vi "Read (Transient).vi"(8 "error in (no error)":errorcluster, 11 "VISA resource name":refnum<visa-resource-name>) -> (0 "error out":errorcluster, 1 "Peak-to-Peak":dbl, 2 "Measurement":dbl, 3 "VISA resource name out":refnum<visa-resource-name>, 5 "Minimum":dbl, 7 "Maximum":dbl)   [LabVIEW 2020, in "Agilent 34401.lvlib"]
doc: "Starts a new single reading and returns the measurement, transient maximum, transient minimum, and peak-to-peak values.\n\n<B>Note:</B>\n\n(1) This VI only applies to the 34410/34411 models. \n\n(2) This VI only supports DC/AC current and voltage measurements."
uses:
  <instrlib>/Agilent 34401/Agilent 34401.lvlib
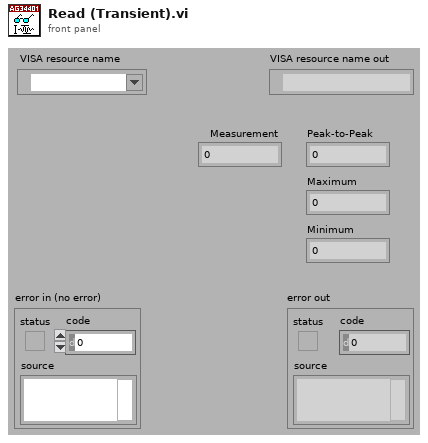
[diagram p1: front panel]
types:
  T1 = typedef "Agilent 34401.lvlib/Extended User Data.ctl" = cluster{"Trigger Source":u16, "Math Storage":u16, "Agilent Model":i32}
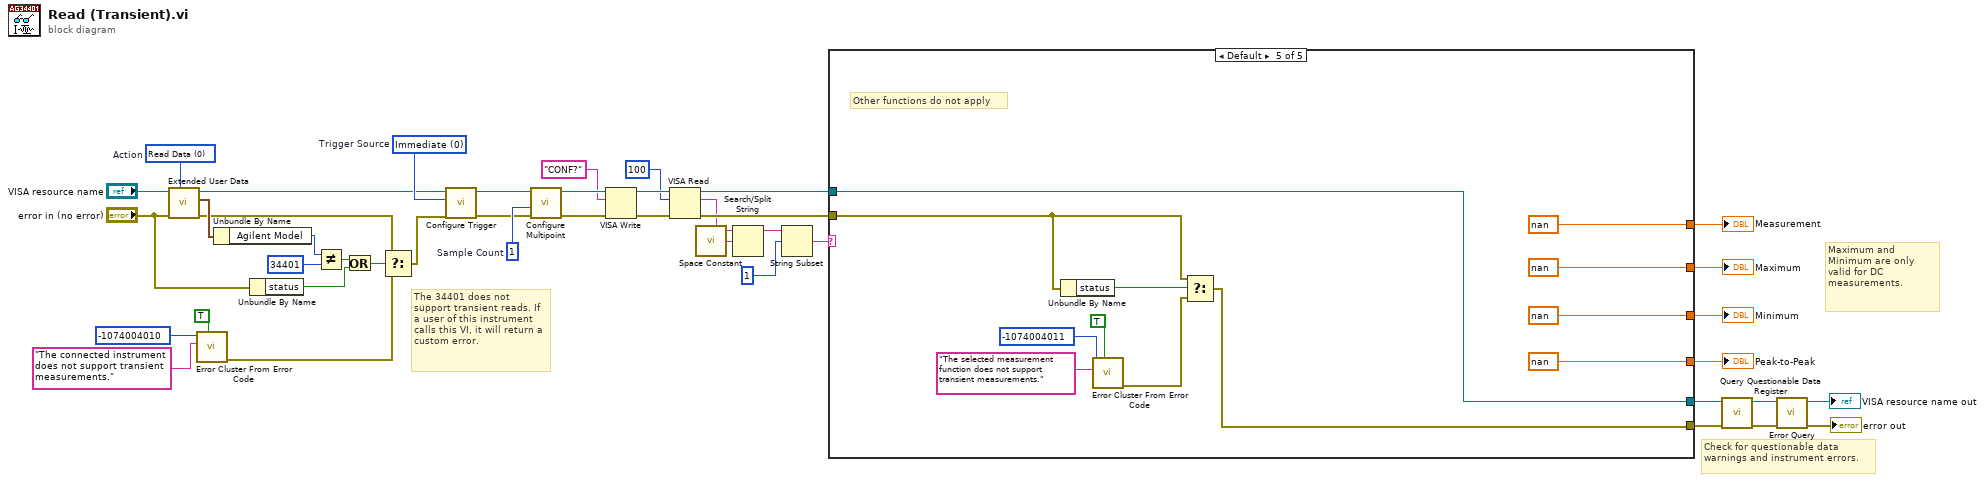
[diagram p0: block diagram]
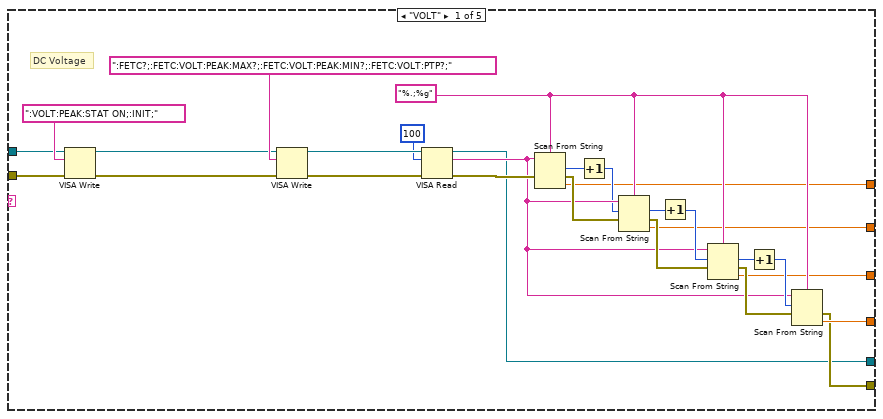
[diagram p2: hidden frame]
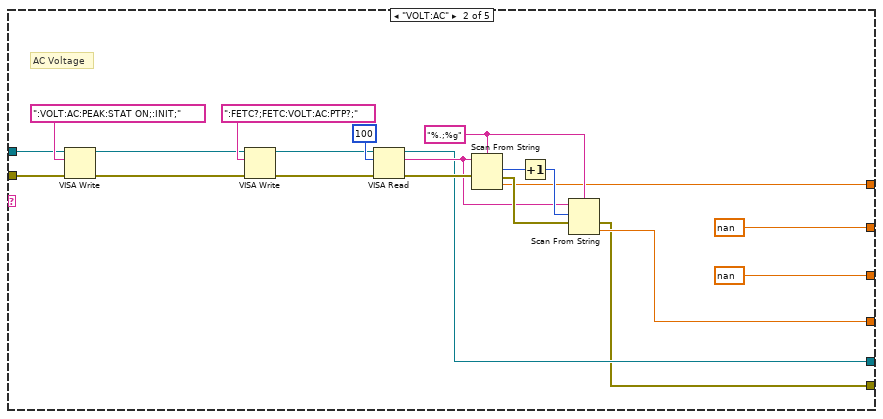
[diagram p3: hidden frame]
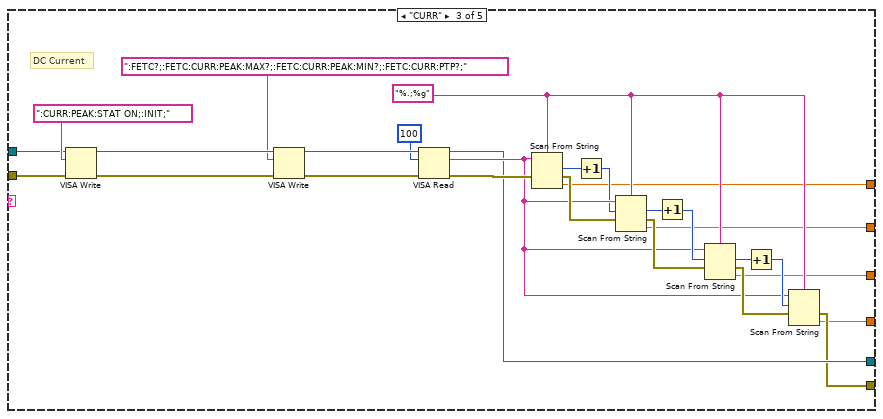
[diagram p4: hidden frame]
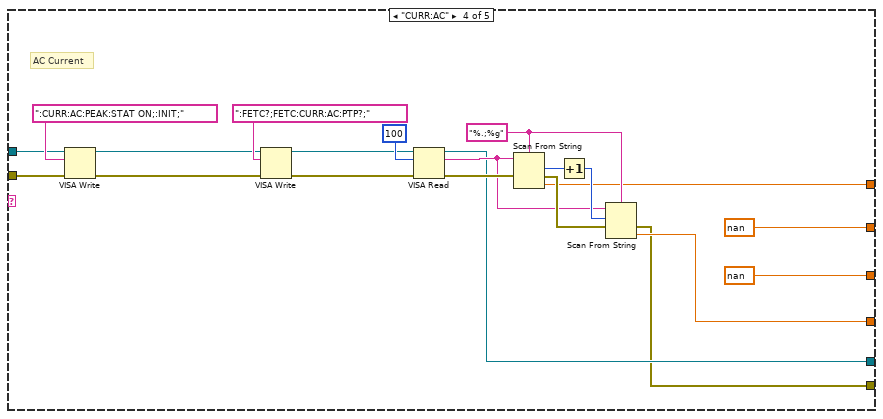
[diagram p5: hidden frame]
diagram:
  w10 = u16 0 items=["Read Data", "Write Data", "Dispose of Data"]  # Action
  w25 = u16 0 items=["Immediate", "Software (Bus)", "External", "Internal"]  # Trigger Source
  w43 = 1  # Sample Count
  # "Check for questionable data warnings and instrument errors."
  # "Maximum and Minimum are only valid for DC measurements."
  # "The 34401 does not support transient reads. If a user of this instrument calls this VI, it will return a custom error."
  n1 = call <instrlib>:"Extended User Data.vi"("Action (0: Read Data)"=w10, "Error In (no error)"="error in (no error)", "VISA resource name in"="VISA resource name") -> ("Error Out"=w9:errorcluster, "User Data Out"=w11:T1, "VISA resource name out"=w5:refnum<visa-resource-name>)  [unwired: 6 in]
  n2 = call <vilib>:"Error Cluster From Error Code.vi"("show call chain? (False)"=TRUE, "error message (\"\")"="The connected instrument does not support transient measurements." ("Source (VI Name)"), "error code (0)"=-1074004010 ("Code")) -> ("error out"=w30:errorcluster)  [unwired: 6 in]
  n3 = Unbundle By Name(w11) -> ("Agilent Model"=w6:i32)
  n4 = Unbundle By Name("error in (no error)") -> ("status"=w27:bool)
  n5 = Not Equal?(x=w6, y=u32 34401 ("x")) -> (x != y?=w28:bool)
  n6 = Or(x=w28, y=w27) -> (x .or. y?=w26:bool)
  n7 = Select(t=w9, s=w26, f=w30) -> (s? t:f=w29:errorcluster)
  n8 = call <instrlib>:"Configure Trigger.vi"("error in (no error)"=w29, "Trigger Source (0: Immediate)"=w25, "VISA resource name"=w5) -> ("error out"=w41:errorcluster, "VISA resource name out"=w42:refnum<visa-resource-name>)  [unwired: 7 in]
  n9 = call <instrlib>:"Configure Multipoint.vi"("error in (no error)"=w41, "Sample Count (1)"=w43, "VISA resource name"=w42) -> ("error out"=w22:errorcluster, "VISA resource name out"=w21:refnum<visa-resource-name>)  [unwired: 7 in]
  n10 = VISA Write(VISA resource name=w21, write buffer="CONF?", error in (no error)=w22) -> (VISA resource name out=w20:refnum<visa-resource-name>, error out=w23:errorcluster)  [unwired: 1 out]
  n11 = VISA Read(VISA resource name=w20, byte count=u32 100, error in (no error)=w23) -> (VISA resource name out=w19:refnum<visa-resource-name>, read buffer=w15:string, error out=w24:errorcluster)  [unwired: 1 out]
  n12 = call <vilib>:"Space Constant.vi"() -> ("String"=w16:string)
  n13 = Search/Split String(string=w15, search string/char (-)=w16) -> (substring before match=w14:string)  [unwired: 1 in, 2 out]
  n14 = String Subset(string=w14, offset (0)=1 ("length (rest)")) -> (substring=w13:string)  [unwired: 1 in]
  n15 = case shown="Default" w13 {
    tunnel: w24 -> [w50 w72 w93 w126 w141]
    tunnel: w19 -> [w51 w71 w92 w125 w148]
    tunnel: [w48 nan w96 nan nan] -> w40
    tunnel: [w47 nan w97 nan nan] -> w39
    tunnel: [w46 w75 w98 w121 nan] -> w38
    tunnel: [w45 w73 w99 w119 w140] -> w36
    tunnel: [w44 w74 w100 w120 w148] -> w37
    tunnel: [w49 w78 w95 w123 nan ("Measurement")] -> w35
    frame "VOLT" {
      w57 = "%.;%g" ("format string")
      # "DC Voltage"
      # "DC Voltage"
      n16 = VISA Write(VISA resource name=w51, write buffer=":VOLT:PEAK:STAT ON;:INIT;", error in (no error)=w50) -> (VISA resource name out=w58:refnum<visa-resource-name>, error out=w59:errorcluster)  [unwired: 1 out]
      n17 = VISA Write(VISA resource name=w58, write buffer=":FETC?;:FETC:VOLT:PEAK:MAX?;:FETC:VOLT:PEAK:MIN?;:FETC:VOLT:PTP?;", error in (no error)=w59) -> (VISA resource name out=w69:refnum<visa-resource-name>, error out=w67:errorcluster)  [unwired: 1 out]
      n18 = VISA Read(VISA resource name=w69, byte count=u32 100, error in (no error)=w67) -> (VISA resource name out=w44:refnum<visa-resource-name>, read buffer=w54:string, error out=w56:errorcluster)  [unwired: 1 out]
      n19 = Scan From String(format string=w57, input string=w54, error in=w56) -> (offset past scan=w53:u32, error out=w55:errorcluster, output 1=w49:dbl)  [unwired: 2 in, 1 out]
      n20 = Increment(x=w53) -> (x+1=w52:u32)
      n21 = Scan From String(format string=w57, input string=w54, initial scan location=w52, error in=w55) -> (offset past scan=w66:u32, error out=w61:errorcluster, output 1=w48:dbl)  [unwired: 1 in, 1 out]
      n22 = Increment(x=w66) -> (x+1=w65:u32)
      n23 = Scan From String(format string=w57, input string=w54, initial scan location=w65, error in=w61) -> (offset past scan=w64:u32, error out=w60:errorcluster, output 1=w47:dbl)  [unwired: 1 in, 1 out]
      n24 = Increment(x=w64) -> (x+1=w63:u32)
      n25 = Scan From String(format string=w57, input string=w54, initial scan location=w63, error in=w60) -> (error out=w45:errorcluster, output 1=w46:dbl)  [unwired: 1 in, 2 out]
    }
    frame "VOLT:AC" {
      w81 = "%.;%g" ("format string")
      # "AC Voltage"
      n26 = VISA Write(VISA resource name=w71, write buffer=":VOLT:AC:PEAK:STAT ON;:INIT;", error in (no error)=w72) -> (VISA resource name out=w85:refnum<visa-resource-name>, error out=w84:errorcluster)  [unwired: 1 out]
      n27 = VISA Write(VISA resource name=w85, write buffer=":FETC?;FETC:VOLT:AC:PTP?;", error in (no error)=w84) -> (VISA resource name out=w89:refnum<visa-resource-name>, error out=w91:errorcluster)  [unwired: 1 out]
      n28 = VISA Read(VISA resource name=w89, byte count=u32 100, error in (no error)=w91) -> (VISA resource name out=w74:refnum<visa-resource-name>, read buffer=w79:string, error out=w86:errorcluster)  [unwired: 1 out]
      n29 = Scan From String(format string=w81, input string=w79, error in=w86) -> (offset past scan=w83:u32, error out=w80:errorcluster, output 1=w78:dbl)  [unwired: 2 in, 1 out]
      n30 = Increment(x=w83) -> (x+1=w82:u32)
      n31 = Scan From String(format string=w81, input string=w79, initial scan location=w82, error in=w80) -> (error out=w73:errorcluster, output 1=w75:dbl)  [unwired: 1 in, 2 out]
    }
    frame "CURR" {
      w109 = "%.;%g" ("format string")
      # "DC Current"
      n32 = VISA Write(VISA resource name=w92, write buffer=":CURR:PEAK:STAT ON;:INIT;", error in (no error)=w93) -> (VISA resource name out=w102:refnum<visa-resource-name>, error out=w103:errorcluster)  [unwired: 1 out]
      n33 = VISA Write(VISA resource name=w102, write buffer=":FETC?;:FETC:CURR:PEAK:MAX?;:FETC:CURR:PEAK:MIN?;:FETC:CURR:PTP?;", error in (no error)=w103) -> (VISA resource name out=w118:refnum<visa-resource-name>, error out=w116:errorcluster)  [unwired: 1 out]
      n34 = VISA Read(VISA resource name=w118, byte count=u32 100, error in (no error)=w116) -> (VISA resource name out=w100:refnum<visa-resource-name>, read buffer=w106:string, error out=w108:errorcluster)  [unwired: 1 out]
      n35 = Scan From String(format string=w109, input string=w106, error in=w108) -> (offset past scan=w105:u32, error out=w107:errorcluster, output 1=w95:dbl)  [unwired: 2 in, 1 out]
      n36 = Increment(x=w105) -> (x+1=w104:u32)
      n37 = Scan From String(format string=w109, input string=w106, initial scan location=w104, error in=w107) -> (offset past scan=w115:u32, error out=w111:errorcluster, output 1=w96:dbl)  [unwired: 1 in, 1 out]
      n38 = Increment(x=w115) -> (x+1=w114:u32)
      n39 = Scan From String(format string=w109, input string=w106, initial scan location=w114, error in=w111) -> (offset past scan=w113:u32, error out=w110:errorcluster, output 1=w97:dbl)  [unwired: 1 in, 1 out]
      n40 = Increment(x=w113) -> (x+1=w112:u32)
      n41 = Scan From String(format string=w109, input string=w106, initial scan location=w112, error in=w110) -> (error out=w99:errorcluster, output 1=w98:dbl)  [unwired: 1 in, 2 out]
    }
    frame "CURR:AC" {
      w129 = "%.;%g" ("format string")
      # "AC Current"
      n42 = VISA Write(VISA resource name=w125, write buffer=":CURR:AC:PEAK:STAT ON;:INIT;", error in (no error)=w126) -> (VISA resource name out=w132:refnum<visa-resource-name>, error out=w133:errorcluster)  [unwired: 1 out]
      n43 = VISA Write(VISA resource name=w132, write buffer=":FETC?;FETC:CURR:AC:PTP?;", error in (no error)=w133) -> (VISA resource name out=w137:refnum<visa-resource-name>, error out=w139:errorcluster)  [unwired: 1 out]
      n44 = VISA Read(VISA resource name=w137, byte count=u32 100, error in (no error)=w139) -> (VISA resource name out=w120:refnum<visa-resource-name>, read buffer=w127:string, error out=w134:errorcluster)  [unwired: 1 out]
      n45 = Scan From String(format string=w129, input string=w127, error in=w134) -> (offset past scan=w131:u32, error out=w128:errorcluster, output 1=w123:dbl)  [unwired: 2 in, 1 out]
      n46 = Increment(x=w131) -> (x+1=w130:u32)
      n47 = Scan From String(format string=w129, input string=w127, initial scan location=w130, error in=w128) -> (error out=w119:errorcluster, output 1=w121:dbl)  [unwired: 1 in, 2 out]
    }
    frame Default {
      # "Other functions do not apply"
      n48 = Unbundle By Name(w141) -> ("status"=w143:bool)
      n49 = call <vilib>:"Error Cluster From Error Code.vi"("show call chain? (False)"=TRUE, "error message (\"\")"="The selected measurement function does not support transient measurements." ("Source (VI Name)"), "error code (0)"=-1074004011 ("Code")) -> ("error out"=w142:errorcluster)  [unwired: 6 in]
      n50 = Select(t=w141, s=w143, f=w142) -> (s? t:f=w140:errorcluster)
    }
  }
  "Maximum" <- w40
  "Minimum" <- w39
  "Peak-to-Peak" <- w38
  "Measurement" <- w35
  n51 = call <instrlib>:"Query Questionable Data Register.vi"("error in (no error)"=w36, "VISA resource name"=w37) -> ("error out"=w4:errorcluster, "VISA resource name out"=w3:refnum<visa-resource-name>)  [unwired: 7 in, 1 out]
  n52 = call <instrlib>:"Error Query.vi"("error in (no error)"=w4, "VISA resource name"=w3) -> ("error out"=→"error out":errorcluster, "VISA resource name out"=→"VISA resource name out":refnum<visa-resource-name>)  [unwired: 6 in, 2 out]
